vi "Tx.vi"(0 "tx.parameters":T3={"tx.trigger select"=enum."Software", "tx.trigger enable"=FALSE, "tx.trigger sync enable"=FALSE, "tx.stream enable"=[FALSE, FALSE], "tx.software trigger"=FALSE, "tx.reset"=FALSE, "tx.abort"=FALSE, "tx.samples to generate"=0, "tx.data source"=enum."SFP Port 0", "tx.duc parameters"=[{"frequency shift"=0.0, "impairments"={"inline gain I"=0.0, "inline gain Q"=0.0, "cross gain I"=0.0, "cross gain Q"=0.0, "pre-gain offset I"=0.0, "pre-gain offset Q"=0.0, "post-gain offset I"=0.0, "post-gain offset Q"=0.0}, "phase"=0.0, "input sample rate"=0.0, "gain"={"gain I"=0.0, "gain Q"=0.0}, "delay"=0.0}, {"frequency shift"=0.0, "impairments"={"inline gain I"=0.0, "inline gain Q"=0.0, "cross gain I"=0.0, "cross gain Q"=0.0, "pre-gain offset I"=0.0, "pre-gain offset Q"=0.0, "post-gain offset I"=0.0, "post-gain offset Q"=0.0}, "phase"=0.0, "input sample rate"=0.0, "gain"={"gain I"=0.0, "gain Q"=0.0}, "delay"=0.0}]} {"tx.duc parameters"."frequency shift" format="%#.48g"}, 5 "tx.start trigger":bool) -> (4 "tx.status":T2={"tx.state"=enum."Idle", "tx.samples processed"=0, "tx.number of fifo underflows"=0, "tx.number of iq data overflows"=[0, 0], "tx.dsp reset done"=FALSE})   [LabVIEW 2016]
uses:
  Tx Parameters.ctl
  HOST/2954/SubVIs/Start Trigger.ctl
  DUC Parameters.ctl
  <instrlib>/_niInstr/DSP/v1/Shared/Public/IQ Impairments.ctl
  <instrlib>/_niInstr/DSP/v1/Shared/Public/IQ Gain.ctl
  Stream Control State.ctl
  <instrlib>/_niInstr/DSP/v1/Shared/niInstr DSP v1 Shared.lvlib
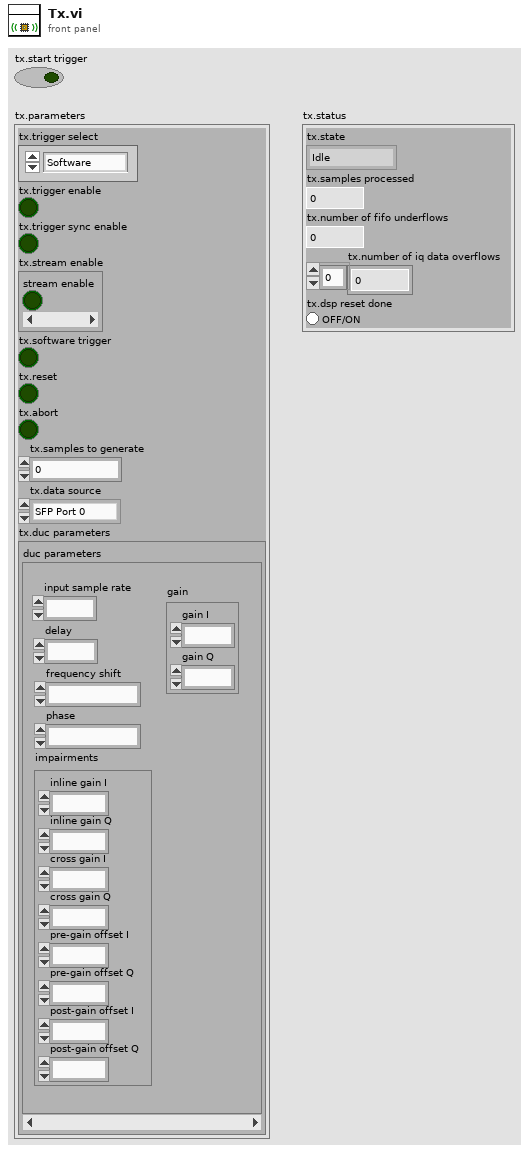
[diagram p1: front panel]
types:
  T1 = typedef "Stream Control State.ctl" = enum16{"Idle", "Active"}
  T2 = cluster{"tx.state":T1, "tx.samples processed":u32, "tx.number of fifo underflows":u32, "tx.number of iq data overflows":u64[], "tx.dsp reset done":bool}
  T3 = typedef "Tx Parameters.ctl" = cluster{"tx.trigger select":T4, "tx.trigger enable":bool, "tx.trigger sync enable":bool, "tx.stream enable":bool[], "tx.software trigger":bool, "tx.reset":bool, "tx.abort":bool, "tx.samples to generate":u32, "tx.data source":enum16{"SFP Port 0", "SFP Port 1", "Host"}, "tx.duc parameters":T5[]}
  T4 = typedef "Start Trigger.ctl" = enum8{"Software", "Digital Edge", "Rx Start Trigger", "Tx Start Trigger", "Immediate", "Future Time Event"}
  T5 = typedef "DUC Parameters.ctl" = cluster{"frequency shift":fxp<+/-,48,0>, "impairments":T6, "phase":fxp<+/-,21,0>, "input sample rate":fxp<+,48,1>, "gain":T7, "delay":fxp<+/-,18,0>}
  T6 = typedef "niInstr DSP v1 Shared.lvlib/IQ Impairments.ctl" = cluster{"inline gain I":fxp<+/-,18,1>, "inline gain Q":fxp<+/-,18,1>, "cross gain I":fxp<+/-,18,1>, "cross gain Q":fxp<+/-,18,1>, "pre-gain offset I":fxp<+/-,18,1>, "pre-gain offset Q":fxp<+/-,18,1>, "post-gain offset I":fxp<+/-,18,1>, "post-gain offset Q":fxp<+/-,18,1>}
  T7 = typedef "niInstr DSP v1 Shared.lvlib/IQ Gain.ctl" = cluster{"gain I":fxp<+/-,24,3>, "gain Q":fxp<+/-,24,3>}
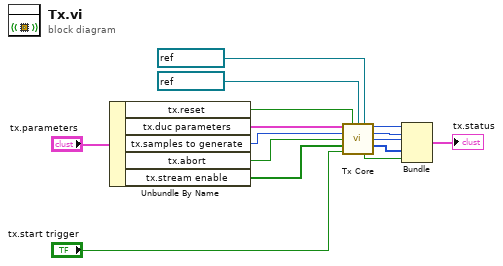
[diagram p0: block diagram]
diagram:
  n1 = Unbundle By Name("tx.parameters") -> ("tx.reset"=w13:bool, "tx.duc parameters"=w14:T5[], "tx.samples to generate"=w12:u32, "tx.abort"=w11:bool, "tx.stream enable"=w1:bool[])
  n2 = call "Tx Core.vi"("duc parameters"=w14, "tx.reset"=w13, "fifo 0"=refnum<k21> "tx 1.fifo", "fifo 1"=refnum<k21> "tx 0.fifo", "tx.samples to generate"=w12, "tx.abort"=w11, "tx.stream enable"=w1, "tx.start trigger"="tx.start trigger") -> ("tx.state"=w9:T1, "tx.samples processed"=w8:u32, "tx.number of fifo underflows"=w7:u32, "tx.number of iq data overflows"=w6:u64[], "tx.dsp reset done"=w5:bool)  [unwired: 3 in]
  n3 = Bundle("tx.state"=w9, "tx.samples processed"=w8, "tx.number of fifo underflows"=w7, "tx.number of iq data overflows"=w6, "tx.dsp reset done"=w5) -> (→"tx.status":T2)  [unwired: 1 in]
